vi "q3w4.vi"() -> ()   [LabVIEW 2021]
panel:
  in  "THETA":dbl
  out "REACTIVE POWER":dbl
  out "ACTIVE POWER":dbl
  out "APPARENT POWER":dbl
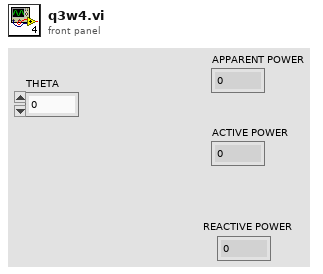
[diagram p1: front panel]
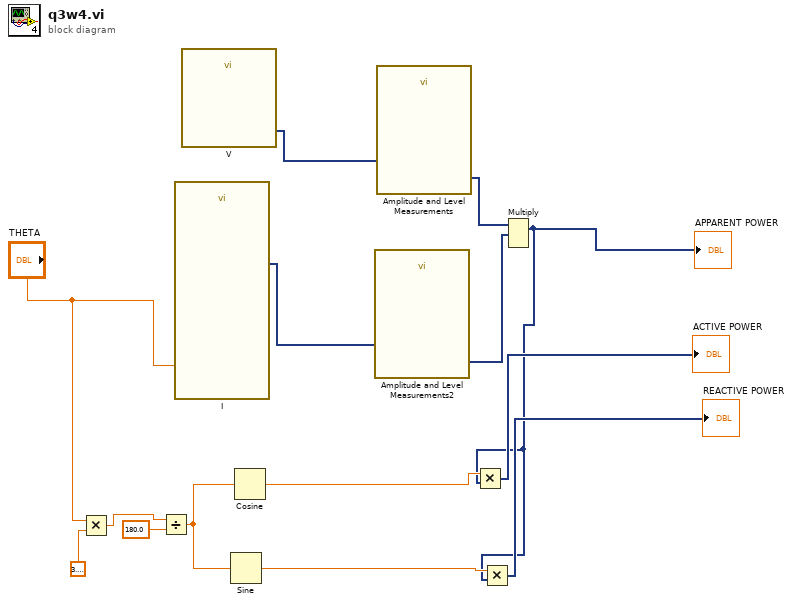
[diagram p0: block diagram]
diagram:
  n1 = Multiply(x="THETA", y=3.141592653589793) -> (x*y=w14:dbl)
  n2 = Divide(x=w14, y=180.0) -> (x/y=w10:dbl)
  n3 = call "I"("Phase"="THETA") -> ("Sine"=w11:dynamicdata)  [unwired: 13 in, 1 out]
  n4 = call "V"() -> ("Sine"=w12:dynamicdata)  [unwired: 14 in, 1 out]
  n5 = Sine(x=w10) -> (sin(x)=w6:dbl)
  n6 = Cosine(x=w10) -> (cos(x)=w7:dbl)
  n7 = call "Amplitude and Level Measurements2"("Signals"=w11) -> ("RMS"=w8:dynamicdata)  [unwired: 13 in, 1 out]
  n8 = call "Amplitude and Level Measurements"("Signals"=w12) -> ("RMS"=w9:dynamicdata)  [unwired: 13 in, 1 out]
  n9 = Multiply(1:w8, 2:w9) -> (0:w3:dynamicdata)  [unwired: 1 in, 1 out]
  "APPARENT POWER" <- w3
  n10 = Multiply(x=w7, y=w3) -> (x*y=→"ACTIVE POWER":dynamicdata)
  n11 = Multiply(x=w6, y=w3) -> (x*y=→"REACTIVE POWER":dynamicdata)
